vi "Port Number to Stream Number.vi"(0 "Port":T1 items=["Port 0", "Port 1", "Port 2", "Port 3"]) -> (4 "Port Out":T1 items=["Port 0", "Port 1", "Port 2", "Port 3"], 6 "rx stream index":i32, 8 "tx stream index":i32)   [LabVIEW 2016, in "Aurora Stream (NI 6592R) (Host).lvlib"]
doc: "Translates the physical port number to the stream numbers associated with that port. Each port has both a TX stream and an RX stream. The appropriate values are provided on <b>rx stream index</b> and <b>tx stream index</b>\n\n<B>Input Parameters</B>\n\n<B>Port</B> The physical port to identify the stream numbers.\n\n<B>Output Parameters</B>\n\n<B>rx stream index</B> The stream index needed for the niInstr Streaming library to talk to the RX port.\n\n<B>tx stream index</B> The stream index needed for the niInstr Streaming library to talk to the TX port."
uses:
  Aurora Stream (NI 6592R) (Host).lvlib
  Port.ctl
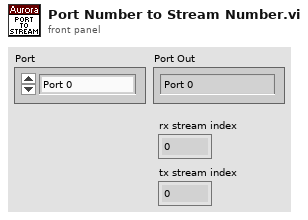
[diagram p1: front panel]
types:
  T1 = typedef "Aurora Stream (NI 6592R) (Host).lvlib/Port.ctl" = i32
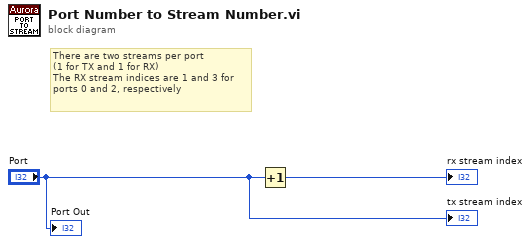
[diagram p0: block diagram]
diagram:
  # "There are two streams per port\n(1 for TX and 1 for RX)\nThe RX stream indices are 1 and 3 for ports 0 and 2, respectively"
  n1 = Increment(x="Port") -> (x+1=→"rx stream index":T1)
  "Port Out" <- "Port"
  "tx stream index" <- "Port"
